vi "Ancestor Classes.vi"(8 "error in (no error)":errorcluster, 11 "Section 1 in":refnum<class "Section 1.lvclass">) -> (0 "error out":errorcluster, 1 "Ancestor Classes":string[](array[string]), 2 "Ancestor Class Pathes":path[](array[path]), 3 "Section 1 out":refnum<class "Section 1.lvclass">)   [LabVIEW 2014, in "LVOOP Introduction.lvlib" / "Section 1.lvclass"]
doc: "This VI returns array of all ancestor classes and their pathes."
uses:
  Section 1.lvclass
  Configuration/Classes/Section/Section.lvclass
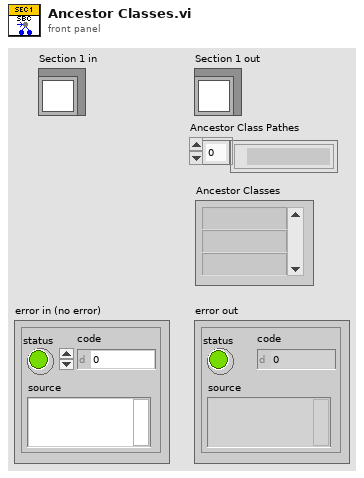
[diagram p1: front panel]
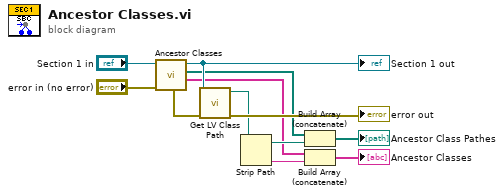
[diagram p0: block diagram]
diagram:
  n1 = call-parent "Ancestor Classes.vi"("error in (no error)"="error in (no error)", "Section in"="Section 1 in") -> ("error out"=w4:errorcluster, "Ancestor Classes"=w1:string[], "Ancestor Class Pathes"=w2:path[], "Section out"=w11:refnum<class "Section 1.lvclass">)  [unwired: 6 in]
  "Section 1 out" <- w11
  n2 = call <vilib>:"Get LV Class Path.vi"("error in (no error)"=w4, "object"=w11) -> ("error out"=→"error out":errorcluster, "class path"=w3:path)  [unwired: 8 in]
  n3 = Strip Path(path=w3) -> (stripped path=w5:path, name=w6:string)
  n4 = Build Array (concatenate)(w2, w5) -> (→"Ancestor Class Pathes":path[])
  n5 = Build Array (concatenate)(w1, w6) -> (→"Ancestor Classes":string[])
